vi "Read Meas.vi"(0 "VISA resource name":refnum<visa-resource-name>, 7 "timeout ms (25000)":u32=25000, 11 "error in (no error)":errorcluster) -> (4 "VISA resource name out":refnum<visa-resource-name>, 6 "Voltage (Volts)":dbl format="%.3f", 8 "Current (Amps)":dbl format="%.3f", 15 "error out":errorcluster)   [LabVIEW 2012, in "Agilent 66XX Series.lvlib"]
doc: "This vi returns the values of the voltage and current displayed on the power supply front panel. The values are measured in Volts and Amps respectively."
uses:
  <instrlib>/Agilent 66XX Series/Agilent 66XX Series.lvlib
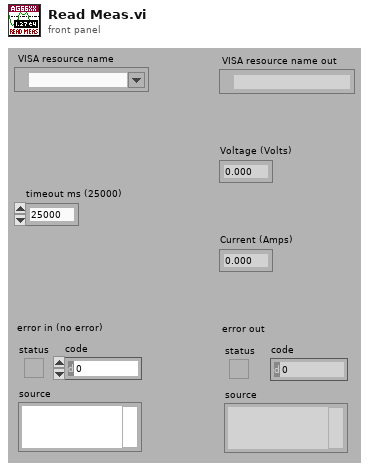
[diagram p1: front panel]
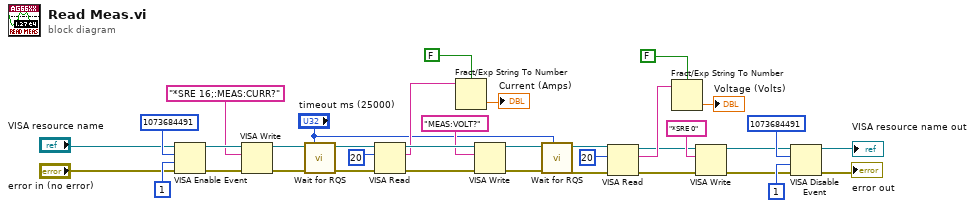
[diagram p0: block diagram]
diagram:
  n1 = VISA Enable Event(8:"error in (no error)", 9:u16 1, 10:u32 1073684491, 11:"VISA resource name") -> (0:w12:errorcluster, 3:w13:refnum<visa-resource-name>)
  n2 = VISA Write(VISA resource name=w13, write buffer="*SRE 16;:MEAS:CURR?", error in (no error)=w12) -> (VISA resource name out=w27:refnum<visa-resource-name>, error out=w25:errorcluster)  [unwired: 1 out]
  n3 = call <vilib>:"Wait for RQS.VI"("timeout (25000 ms)"="timeout ms (25000)", "error in (no error)"=w25, "VISA resource name"=w27) -> ("error out"=w24:errorcluster, "VISA resource name out"=w26:refnum<visa-resource-name>)  [unwired: 6 in, 1 out]
  n4 = VISA Read(VISA resource name=w26, byte count=20, error in (no error)=w24) -> (VISA resource name out=w35:refnum<visa-resource-name>, read buffer=w31:string, error out=w34:errorcluster)  [unwired: 1 out]
  n5 = Fract/Exp String To Number(use system decimal point (T)=FALSE, string=w31) -> (number=→"Current (Amps)":dbl)  [unwired: 2 in, 1 out]
  n6 = VISA Write(VISA resource name=w35, write buffer="MEAS:VOLT?", error in (no error)=w34) -> (VISA resource name out=w22:refnum<visa-resource-name>, error out=w21:errorcluster)  [unwired: 1 out]
  n7 = call <vilib>:"Wait for RQS.VI"("timeout (25000 ms)"="timeout ms (25000)", "error in (no error)"=w21, "VISA resource name"=w22) -> ("error out"=w20:errorcluster, "VISA resource name out"=w19:refnum<visa-resource-name>)  [unwired: 6 in, 1 out]
  n8 = VISA Read(VISA resource name=w19, byte count=u32 20, error in (no error)=w20) -> (VISA resource name out=w17:refnum<visa-resource-name>, read buffer=w30:string, error out=w16:errorcluster)  [unwired: 1 out]
  n9 = Fract/Exp String To Number(use system decimal point (T)=FALSE, string=w30) -> (number=→"Voltage (Volts)":dbl)  [unwired: 2 in, 1 out]
  n10 = VISA Write(VISA resource name=w17, write buffer="*SRE 0", error in (no error)=w16) -> (VISA resource name out=w3:refnum<visa-resource-name>, error out=w6:errorcluster)  [unwired: 1 out]
  n11 = VISA Disable Event(8:w6, 9:u16 1, 10:u32 1073684491, 11:w3) -> (0:→"error out":errorcluster, 3:→"VISA resource name out":refnum<visa-resource-name>)
